vi "CTR_XML-parse.vi"(8 "error in":errorcluster, 11 "DOM document in":refnum<k20>) -> (0 "error out":errorcluster={"status"=TRUE, "code"=0, "source"=""}, 2 "channel Definitions out":T1, 3 "DOM document out":refnum<k20>)   [LabVIEW 2024]
uses:
  Control/CTR_channelDefinitions.ctl
  10f0a1c7-9ed0-4649-ba5a-dd6b15093da3.vi
  0a0fd023-9856-4cf8-bcff-a165bffb7d59.vi
  <vilib>/xml/Close Reference(Node).vi
  <vilib>/Utility/error.llb/Error Cluster From Error Code.vi
  <vilib>/ErrorRing/Error Ring.xnode
  <vilib>/Comparison/Less/Less Functor/Less Functor.lvclass
  <vilib>/xml/NI_XML.lvlib
  <resource>/objmgr/DOMUserDefRef.rc
panel:
  in  "channel Definitions":T1
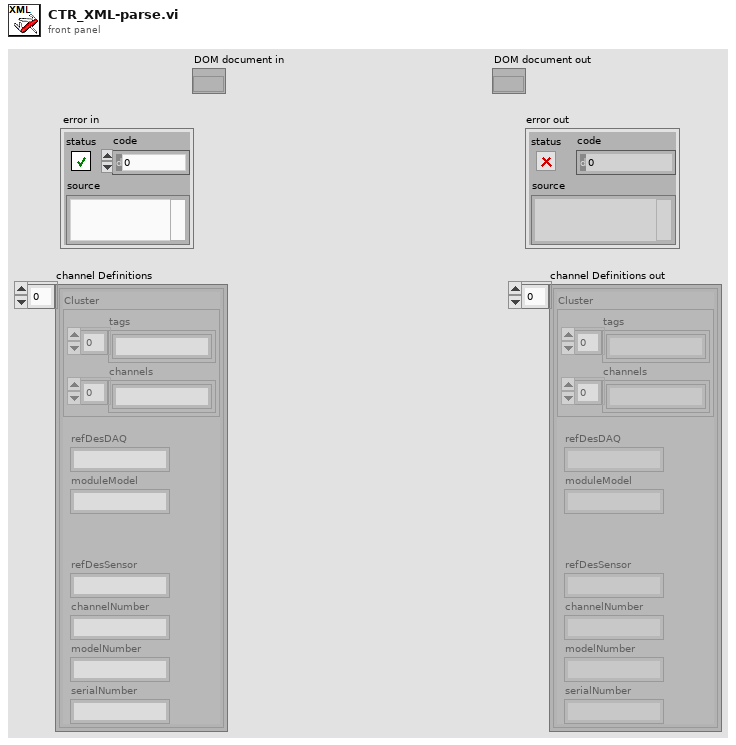
[diagram p1: front panel]
types:
  T1 = typedef "CTR_channelDefinitions.ctl" = cluster{"refDesDAQ":string, "moduleModel":string, "refDesSensor":string, "channelNumber":string, "modelNumber":string, "serialNumber":string, "Cluster":cluster{"tags":string[], "channels":string[]}}[]
  T2 = cluster{"[0]":string, "[1]":string, "[2]":string, "[3]":string, "[4]":string, "[5]":string}
  T3 = cluster{"refDesDAQ":string, "moduleModel":string, "refDesSensor":string, "channelNumber":string, "modelNumber":string, "serialNumber":string, "Cluster":cluster{"tags":string[], "channels":string[]}}
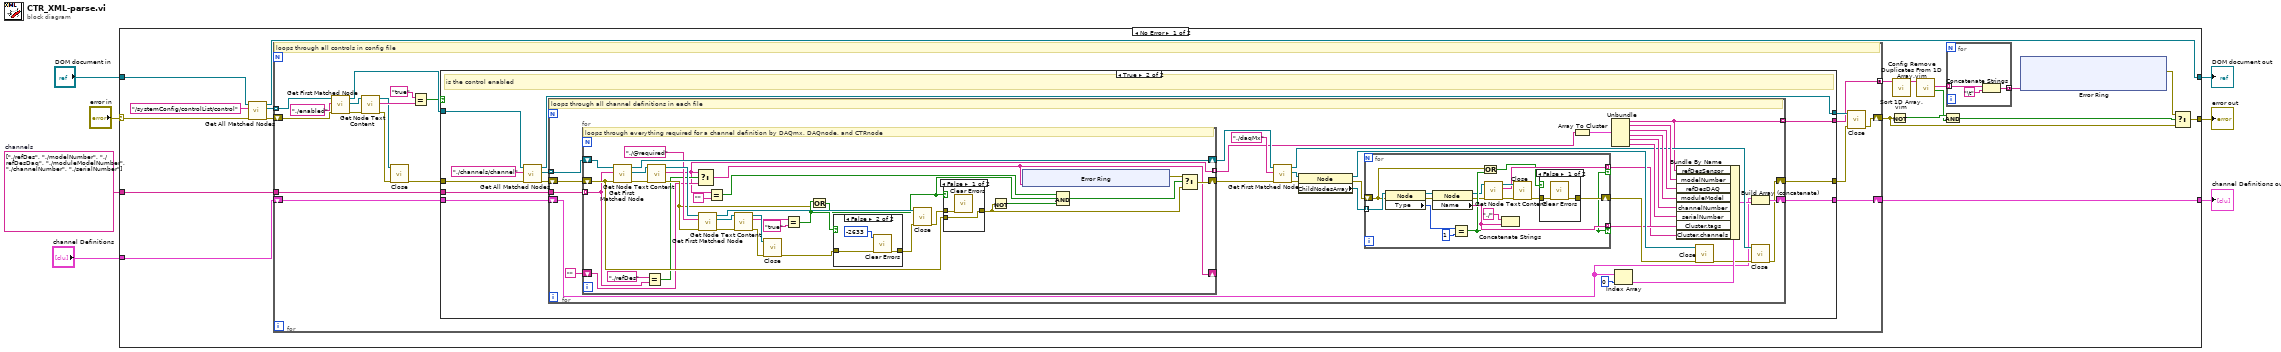
[diagram p0: block diagram]
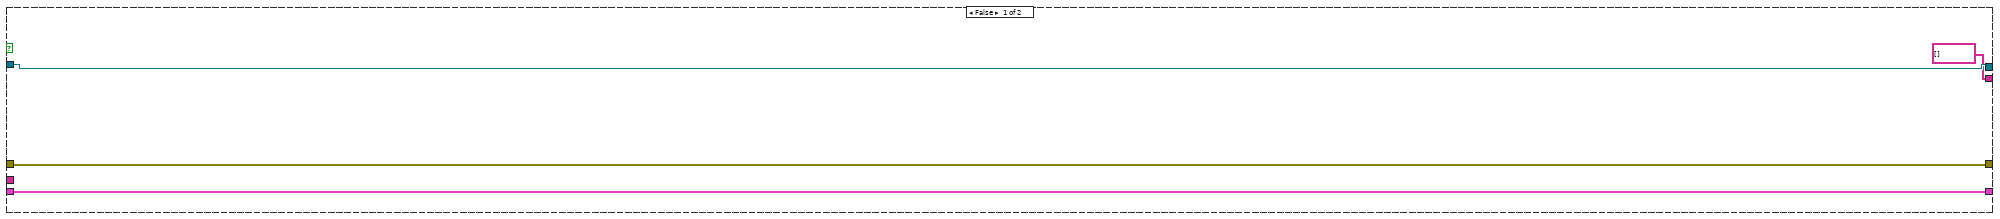
[diagram p2: hidden frame]
diagram:
  w4 = string[] ["./refDes", "./modelNumber", "./refDesDaq", "./moduleModelNumber", "./channelNumber", "./serialNumber"]  # channels
  n1 = case shown="No Error" "error in" {
    selector: "error in" -> [w25 w171]
    tunnel: [w13 w171] -> w6
    tunnel: [w21 w170] -> w5
    tunnel: "DOM document in" -> [w26 w170]
    tunnel: "channel Definitions" -> [w20 w169]
    tunnel: w4 -> [w19 _]
    tunnel: [w18 w169] -> w2
    frame No Error {
      n2 = call <vilib>:"Get All Matched Nodes.vi"("error in (no error)"=w25, "XPath expression"="/systemConfig/controlList/control", "node in"=w26) -> ("error out"=w22:errorcluster, "node result array"=w23:refnum<k20>[], "node out"=w21:refnum<k20>)  [unwired: 6 in]
      n3 = for {
        tunnel: w23 -> [w44] mode=indexing
        shift-right: [w53] -> w14
        shift-left: w22 -> [w47]
        tunnel: w19 -> [w50]
        shift-right: [w51] -> w18
        shift-left: w20 -> [w52]
        tunnel: [w37] -> w17 mode=concatenating
        # "loops through all controls in config file"
        n4 = call <vilib>:"Get First Matched Node.vi"("error in (no error)"=w47, "XPath expression"="./enabled", "node in"=w44) -> ("error out"=w48:errorcluster, "node result"=w42:refnum<k20>, "node out"=w45:refnum<k20>)  [unwired: 6 in]
        n5 = call <vilib>:"Get Node Text Content.vi"("error in (no error)"=w48, "node in"=w42) -> ("error out"=w49:errorcluster, "node text"=w40:string, "node out"=w39:refnum<k20>)  [unwired: 7 in]
        n6 = call-poly <vilib>:"Close.vi"("error in (no error)"=w49, "node"=w39) -> ("error out"=w46:errorcluster)  [unwired: 7 in]
        n7 = Equal?(x="true", y=w40) -> (x = y?=w41:bool)
        n8 = case shown="True" w41 {
          tunnel: w46 -> [w58 w70]
          tunnel: w45 -> [w59 w69]
          tunnel: [w58 w65] -> w55
          tunnel: [w59 w64] -> w54
          tunnel: w52 -> [w57 w63]
          tunnel: [w57 w62] -> w51
          tunnel: w50 -> [_ w61]
          tunnel: [string[] [] w60] -> w37
          frame False {
          }
          frame True {
            # "is the control enabled"
            n9 = call <vilib>:"Get All Matched Nodes.vi"("error in (no error)"=w70, "XPath expression"="./channels/channel", "node in"=w69) -> ("error out"=w67:errorcluster, "node result array"=w66:refnum<k20>[], "node out"=w64:refnum<k20>)  [unwired: 6 in]
            n10 = for {
              shift-right: [w89] -> w65
              shift-left: w67 -> [w98]
              tunnel: w66 -> [w101] mode=indexing
              tunnel: w61 -> [w85]
              shift-right: [w99] -> w62
              shift-left: w63 -> [w82]
              tunnel: [w80] -> w60 mode=indexing
              # "loops through all channel definitions in each file"
              n11 = for {
                shift-right: [w151] -> w87
                shift-left: w101 -> [w154]
                tunnel: w85 -> [w126] mode=indexing
                shift-right: [w136] -> w86
                shift-left: w98 -> [w132]
                tunnel: [w123] -> w79 mode=indexing
                shift-right: [w122] -> _
                shift-left: "" -> [w124]
                # "loops through everything required for a channel definition by DAQmx, DAQnode, and CTRnode"
                n12 = call <vilib>:"Get First Matched Node.vi"("error in (no error)"=w132, "XPath expression"=w126, "node in"=w154) -> ("error out"=w153:errorcluster, "node result"=w152:refnum<k20>, "node out"=w151:refnum<k20>)  [unwired: 6 in]
                n13 = Equal?(x="./refDes", y=w126) -> (x = y?=w125:bool)
                n14 = call <vilib>:"Get Node Text Content.vi"("error in (no error)"=w153, "node in"=w152) -> ("error out"=w128:errorcluster, "node text"=w123:string, "node out"=w150:refnum<k20>)  [unwired: 7 in]
                n15 = Select(t=w123, s=w125, f=w124) -> (s? t:f=w122:string)
                n16 = call <vilib>:"Get First Matched Node.vi"("error in (no error)"=w128, "XPath expression"="./@required" ("string"), "node in"=w150) -> ("error out"=w149:errorcluster, "node result"=w148:refnum<k20>, "node out"=w147:refnum<k20>)  [unwired: 6 in]
                n17 = Equal?(x=w123, y="") -> (x = y?=w140:bool)
                n18 = call <vilib>:"Get Node Text Content.vi"("error in (no error)"=w149, "node in"=w148) -> ("error out"=w146:errorcluster, "node text"=w143:string, "node out"=w145:refnum<k20>)  [unwired: 7 in]
                n19 = call-poly <vilib>:"Close.vi"("error in (no error)"=w146, "node"=w145) -> ("error out"=w134:errorcluster)  [unwired: 7 in]
                n20 = Equal?(x=w143, y="true") -> (x = y?=w129:bool)
                n21 = Or(x=w129, y=w128) -> (x .or. y?=w130:bool)
                n22 = case shown="False" w130 {
                  tunnel: [w158 w160] -> w135
                  tunnel: w134 -> [w158 w159]
                  frame True {
                  }
                  frame False {
                    n23 = call <vilib>:"Clear Errors.vi"("error in (no error)"=w159, "specific error code to clear (0: all)"=-2633) -> ("error out"=w160:errorcluster)  [unwired: 4 in, 1 out]
                  }
                }
                n24 = call-poly <vilib>:"Close.vi"("error in (no error)"=w135, "node"=w147) -> ("error out"=w133:errorcluster)  [unwired: 7 in]
                n25 = case shown="False" w129 {
                  tunnel: w133 -> [w156 w157]
                  tunnel: w132 -> [w155 _]
                  tunnel: [w155 w157] -> w131
                  frame False {
                    n26 = call <vilib>:"Clear Errors.vi"("error in (no error)"=w156) -> ()  [unwired: 5 in, 2 out]
                  }
                  frame True {
                  }
                }
                n27 = Not(x=w131) -> (.not. x?=w139:bool)
                n28 = xnode "Error Ring"("parameter 0"=w122) -> ("error out"=w137:errorcluster)
                n29 = Compound Arithmetic op=AND(w140, w129, w139) -> (w138:bool)
                n30 = Select(t=w137, s=w138, f=w131) -> (s? t:f=w136:errorcluster)
              }
              n31 = call <vilib>:"Get First Matched Node.vi"("error in (no error)"=w86, "XPath expression"="./daqMx", "node in"=w87) -> ("error out"=w74:errorcluster, "node result"=w78:refnum<k20>, "node out"=w88:refnum<k20>)  [unwired: 6 in]
              n32 = property class="Node"(reference=w78, error in=w74) -> (reference out=w76:refnum<k20>, error out=w73:errorcluster, "ChildNodesArray"=w77:refnum<k20>[])
              n33 = for {
                tunnel: w77 -> [w116] mode=indexing
                shift-right: [w108] -> w75
                shift-left: w73 -> [w105]
                tunnel: [w111] -> w72 mode=indexing if=w106
                tunnel: [w112] -> w71 mode=indexing if=w106
                n34 = property class="Node"(reference=w116, error in=w105) -> (reference out=w118:refnum<k20>, error out=w117:errorcluster, "Type"=w110:i32)
                n35 = property class="Node"(reference=w118, error in=w117) -> (reference out=w103:refnum<k20>, error out=w104:errorcluster, "Name"=w111:string)
                n36 = Equal?(x=w110, y=1) -> (x = y?=w106:bool)
                n37 = Or(x=w105, y=w106) -> (x .or. y?=w107:bool)
                n38 = call <vilib>:"Get Node Text Content.vi"("error in (no error)"=w104, "node in"=w103) -> ("error out"=w114:errorcluster, "node text"=w112:string, "node out"=w113:refnum<k20>)  [unwired: 7 in]
                n39 = Concatenate Strings("./" ("string"), w111) -> ()  [unwired: 1 out]
                n40 = call-poly <vilib>:"Close.vi"("error in (no error)"=w114, "node"=w113) -> ("error out"=w102:errorcluster)  [unwired: 7 in]
                n41 = case shown="False" w107 {
                  tunnel: w102 -> [w120 w121]
                  tunnel: [w119 w121] -> w108
                  frame False {
                    n42 = call <vilib>:"Clear Errors.vi"("error in (no error)"=w120) -> ("error out"=w119:errorcluster)  [unwired: 5 in, 1 out]
                  }
                  frame True {
                  }
                }
              }
              n43 = Array To Cluster(array=w79) -> (cluster=w95:T2)
              n44 = Unbundle(w95) -> ("[0]"=w80:string, "[1]"=w94:string, "[2]"=w93:string, "[3]"=w92:string, "[4]"=w91:string, "[5]"=w90:string)
              n45 = Index Array(array=w82, index=0) -> (element=w97:T3)
              n46 = Bundle By Name(cluster=w97, "refDesSensor"=w80, "modelNumber"=w94, "refDesDAQ"=w93, "moduleModel"=w92, "channelNumber"=w91, "serialNumber"=w90, "Cluster.tags"=w72, "Cluster.channels"=w71) -> (w83:T3)
              n47 = call-poly <vilib>:"Close.vi"("error in (no error)"=w75, "node"=w76) -> ("error out"=w96:errorcluster)  [unwired: 7 in]
              n48 = Build Array (concatenate)(w82, w83) -> (w99:T1)
              n49 = call-poly <vilib>:"Close.vi"("error in (no error)"=w96, "node"=w88) -> ("error out"=w89:errorcluster)  [unwired: 7 in]
            }
          }
        }
        n50 = call-poly <vilib>:"Close.vi"("error in (no error)"=w55, "node"=w54) -> ("error out"=w53:errorcluster)  [unwired: 7 in]
      }
      n51 = Not(x=w14) -> (.not. x?=w15:bool)
      n52 = call "Sort 1D Array.vim"("unsorted array"=w17) -> ("sorted array"=w10:string[])  [unwired: 10 in]
      n53 = call "Config Remove Duplicates From 1D Array.vim"("array"=w10) -> ("duplicates?"=w9:bool, "array of duplicates"=w8:string[])  [unwired: 8 in, 1 out]
      n54 = And(x=w15, y=w9) -> (x .and. y?=w16:bool)
      n55 = for {
        tunnel: w8 -> [w29] mode=indexing
        tunnel: [w27] -> w11 mode=concatenating
        n56 = Concatenate Strings(w29, "\t") -> (w27:string)
      }
      n57 = xnode "Error Ring"("parameter 0"=w11) -> ("error out"=w12:errorcluster)
      n58 = Select(t=w12, s=w16, f=w14) -> (s? t:f=w13:errorcluster)
    }
    frame Error {
    }
  }
  "error out" <- w6
  "DOM document out" <- w5
  "channel Definitions out" <- w2
